vi "Line Configuration Dialog.vi"(8 "error in":errorcluster, 9 "engine configuration in":refnum<class "engine configuration.lvclass">, 10 "tag bus configurable plugin module configuration":refnum<class "PID Module 2 configuration.lvclass">, 11 "Line":T3) -> (0 "error out":errorcluster, 1 "success":bool, 2 "changed":bool, 3 "Mappings out":T2)   [LabVIEW 2015, in "PID Module 2 editor node.lvclass"]
doc: "A dialog for allowing a user to specify the values of a new line."
uses:
  PID Module 2 editor node.lvclass
  module/configuration/Line.ctl
  <vilib>/NI/Tag Bus Module Framework/channel/TBM channel.lvclass
  Mappings.ctl
  Map.ctl
  module/configuration/permissions.ctl
  <vilib>/NI/Module Execution Interface/Engine Configuration/engine configuration.lvclass
  module/configuration/PID Module 2 configuration.lvclass
  <vilib>/NI/Tag Bus/tag/tag descriptor.lvclass/tag descriptor.ctl
  <vilib>/NI/Tag Bus Module Framework/channel/TBM channel.lvclass/TBM channel.ctl
  <vilib>/NI/Configuration Framework/serializable configuration/NISE_CEF_serializable configuration.lvclass/NISE_CEF_serializable configuration.ctl
  <vilib>/NI/Tag Bus/tag/write tag name.vi
  <vilib>/NI/Tag Bus/tag/write data type.vi
  <vilib>/NI/Tag Bus Module Framework/channel/Write channel classification.vi
  <vilib>/NI/Configuration Framework/serializable configuration/Read UID.vi
  <vilib>/NI/Tag Bus/tag/read data type.vi
  <vilib>/NI/Tag Bus Module Framework/channel/Read channel classification.vi
  <vilib>/Utility/LVClass/Get LV Class Name.vi
  <vilib>/NI/Configuration Framework/error generator/NISE_error generator.vi
  <vilib>/NI/Tag Bus/tag/tag descriptor.lvclass
  <vilib>/NI/DCAF UI Toolkit/Controls/DCAF UI Elements.lvlib
panel:
  out "errors":string
  in  "Access Type":T1
  in  "Tag":i32(listbox)
  in  "Data Type":i32(listbox)
  in  "Channel Name":string
  in  "cancel":bool
  in  "ok":bool
  # "#CodeRecommended Add implementation details here. For example, a shared variable URL."
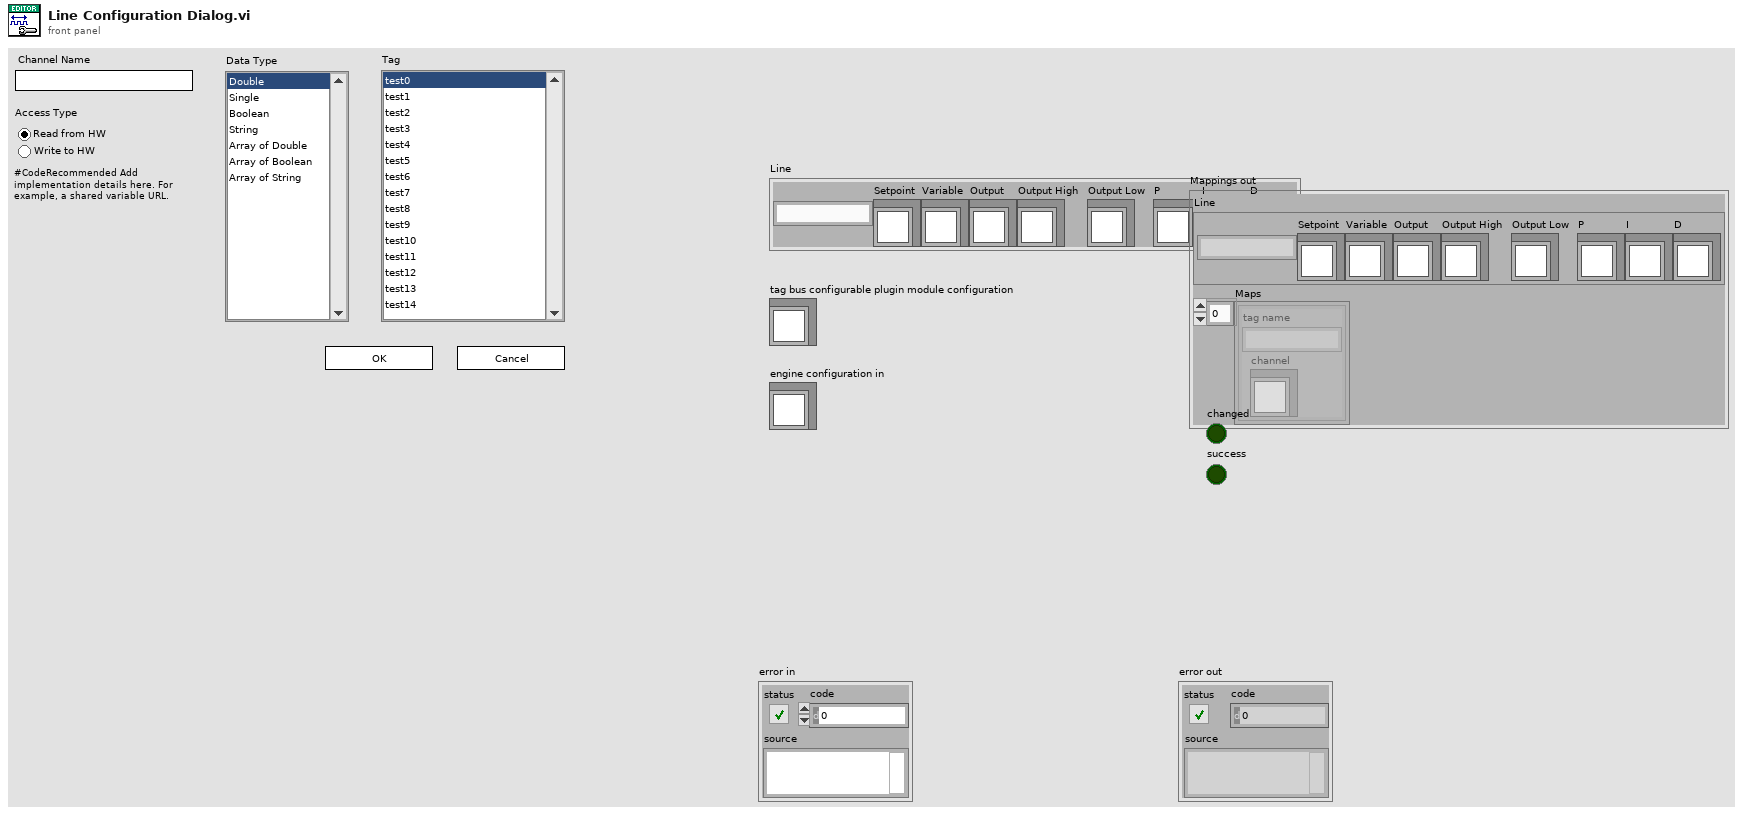
[diagram p1: front panel]
types:
  T1 = typedef "PID Module 2 configuration.lvclass/permissions.ctl" = enum32{"Read from HW", "Write to HW"}
  T2 = typedef "PID Module 2 editor node.lvclass/Mappings.ctl" = cluster{"Line":T3, "Maps":T4[]}
  T3 = typedef "PID Module 2 configuration.lvclass/Line.ctl" = cluster{"PID ID":string, "Setpoint":refnum<class "TBM channel.lvclass">, "Variable":refnum<class "TBM channel.lvclass">, "Output":refnum<class "TBM channel.lvclass">, "Output High":refnum<class "TBM channel.lvclass">, "Output Low":refnum<class "TBM channel.lvclass">, "P":refnum<class "TBM channel.lvclass">, "I":refnum<class "TBM channel.lvclass">, "D":refnum<class "TBM channel.lvclass">}
  T4 = typedef "PID Module 2 editor node.lvclass/Map.ctl" = cluster{"channel":refnum<class "TBM channel.lvclass">, "tag name":string}
  T5 = typedef "tag bus.lvlib/tag descriptor.lvclass/Data Type.ctl" = enum16{"Double", "Single", "I64", "I32", "I16", "I8", "U64", "U32", "U16", "U8", "Boolean", "String", "Array of Double", "Array of Single", "Array of I64", "Array of I32", "Array of I16", "Array of I8", "Array of U64", "Array of U32", "Array of U16", "Array of U8", "Array of Boolean", "Array of String"}
  T6 = typedef "TBM channel.lvclass/channel classification.ctl" = enum16{"input data", "output data", "processing parameter", "processing result"}
  T7 = enum8{"Enabled", "Disabled", "Disabled and Grayed Out"}
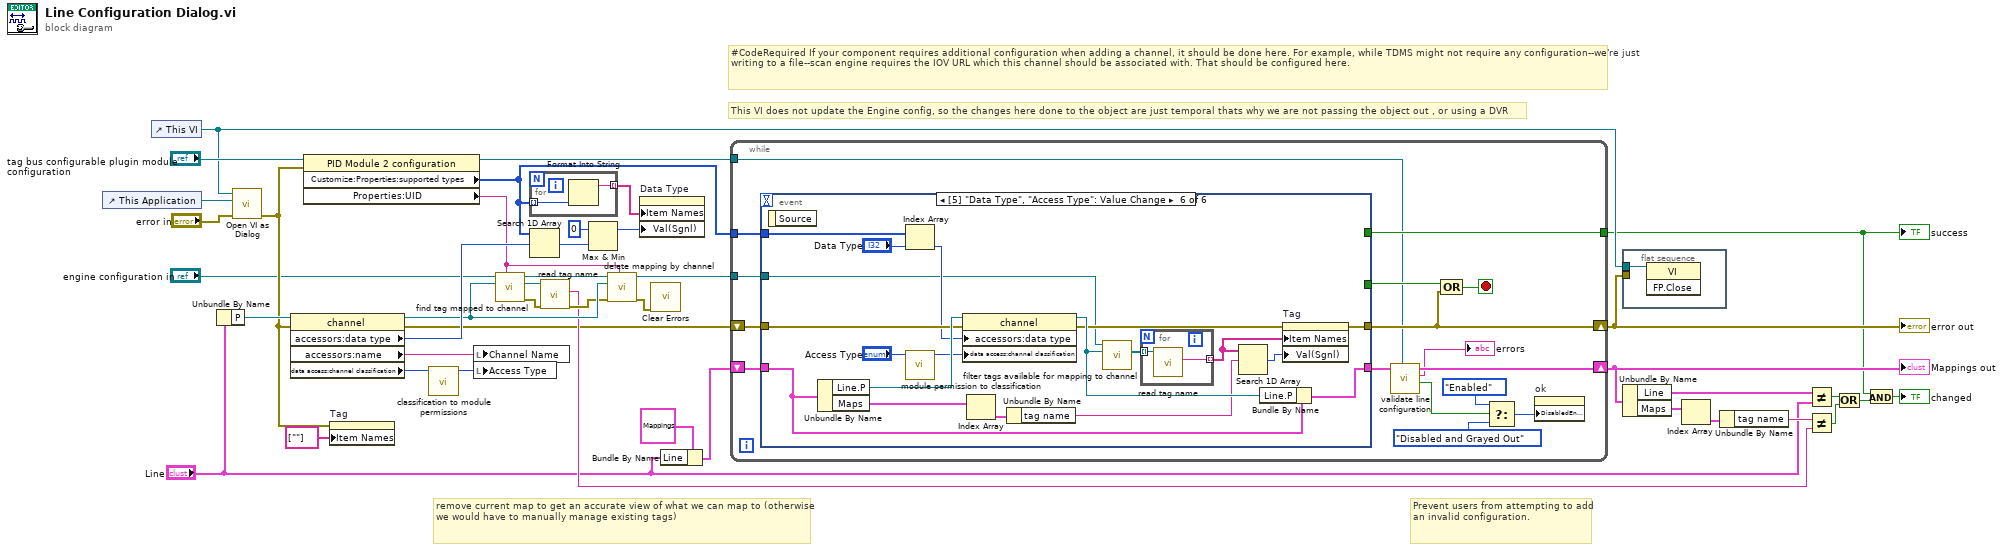
[diagram p0: block diagram]
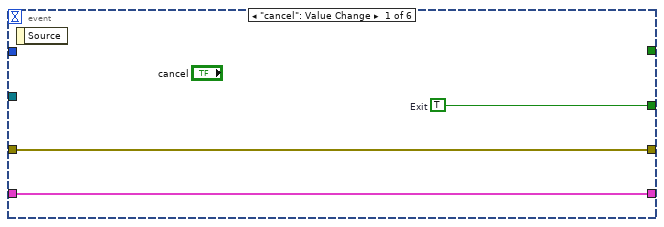
[diagram p2: hidden frame]
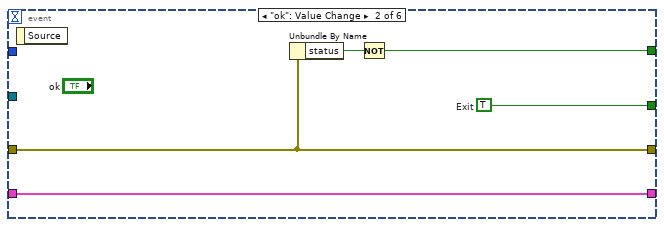
[diagram p3: hidden frame]
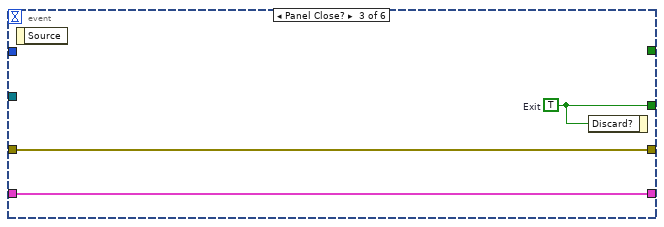
[diagram p4: hidden frame]
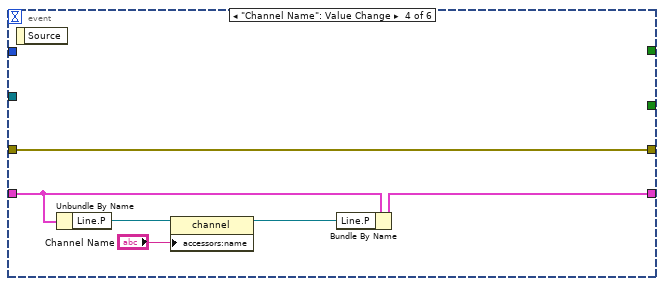
[diagram p5: hidden frame]
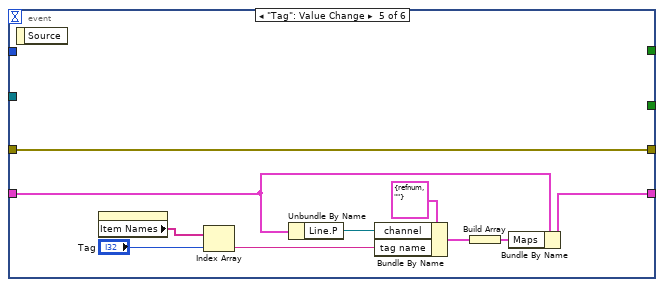
[diagram p6: hidden frame]
diagram:
  # "Prevent users from attempting to add an invalid configuration."
  # "This VI does not update the Engine config, so the changes here done to the object are just temporal thats why we are not passing the object out , or using a DVR"
  # "remove current map to get an accurate view of what we can map to (otherwise we would have to manually manage existing tags)"
  # "#CodeRequired If your component requires additional configuration when adding a channel, it should be done here. For example, while TDMS might not require any configuration--we're just writing to a file--scan engine requires the IOV URL which this channel should be associated with. That should be configured here."
  n1 = control-ref of="This Application"() -> (w31:refnum<vi>)
  n2 = control-ref of="This VI"() -> (w14:refnum<vi>)
  n3 = Unbundle By Name("Line") -> ("P"=w41:refnum<class "TBM channel.lvclass">)
  n4 = call <vilib>:"Open VI as Dialog.vi"("error in (no error)"="error in", "This Application"=w31, "VI in"=w14) -> ("error out"=w29:errorcluster)  [unwired: 8 in]
  n5 = property class="channel"(reference=w41, error in=w29) -> (reference out=w25:refnum<class "TBM channel.lvclass">, error out=w7:errorcluster, "accessors:data type"=w38:T5, "accessors:name"=w6:string, "data access:channel classification"=w8:T6)
  n6 = property class="PID Module 2 configuration"(reference="tag bus configurable plugin module configuration", error in=w29) -> (reference out=w26:refnum<class "PID Module 2 configuration.lvclass">, "Customize:Properties:supported types"=w1:T5[], "Properties:UID"=w9:string)  [unwired: 1 out]
  n7 = property on="Tag" class="LstBox (strict)"(error in=w29, "Item Names"=string[] [""]) -> ()  [unwired: 1 in, 2 out]
  n8 = call "classification to module permissions.vi"("channel classification"=w8) -> ("permissions"=w10:T1)  [unwired: 10 in]
  n9 = local write "Channel Name"(w6) -> ()
  n10 = local write "Access Type"(w10) -> ()
  n11 = call <vilib>:"find tag mapped to channel.vi"("owner"=w9, "channel"=w25, "engine configuration in"="engine configuration in") -> ("error out"=w21:errorcluster, "tag"=w22:refnum<class "tag descriptor.lvclass">, "engine configuration out"=w27:refnum<class "engine configuration.lvclass">)  [unwired: 6 in]
  n12 = for {
    tunnel: w1 -> [w44] mode=indexing
    tunnel: [w43] -> w40 mode=indexing
    n13 = Format Into String(w44) -> (resulting string=w43:string)  [unwired: 3 in, 1 out]
  }
  n14 = Search 1D Array(1D array=w1, element=w38) -> (index of element=w24:i32)  [unwired: 1 in]
  n15 = call <vilib>:"read tag name.vi"("error in"=w21, "system tag in"=w22) -> ("error out"=w20:errorcluster, "name"=w13:string)  [unwired: 7 in, 1 out]
  n16 = Max & Min(x=0 ("f"), y=w24) -> (max(x,y)=w11:i32)  [unwired: 1 out]
  n17 = call <vilib>:"delete mapping by channel.vi"("owner ID"=w9, "error in"=w20, "channel"=w25, "engine configuration in"=w27) -> ("error out"=w37:errorcluster, "engine configuration out"=w42:refnum<class "engine configuration.lvclass">)  [unwired: 6 in]
  n18 = property on="Data Type" class="LstBox (strict)"("Item Names"=w40, "Val(Sgnl)"=w11) -> ()  [unwired: 2 in, 2 out]
  n19 = call <vilib>:"Clear Errors.vi"("error in (no error)"=w37) -> ()  [unwired: 5 in, 2 out]
  n20 = Bundle By Name(cluster=T2 {"Line"={"PID ID"="", "Setpoint"=refnum, "Variable"=refnum, "Output"=refnum, "Output High"=refnum, "Output Low"=refnum, "P"=refnum, "I"=refnum, "D"=refnum}, "Maps"=[]} ("Mappings out"), "Line"="Line") -> (w34:T2)
  n21 = while {
    shift-right: [w52] -> w5
    shift-left: w7 -> [w59]
    tunnel: [w58] -> w4
    shift-right: [w53] -> w32
    shift-left: w34 -> [w55]
    tunnel: w42 -> [w60]
    tunnel: w26 -> [w47]
    tunnel: w1 -> [w46]
    stop <- w56 stop-if-true
    n22 = event shown="[5] \"Data Type\", \"Access Type\": Value Change" {
      selector: _ -> [_ _ _ _ _ _]
      dyn-events: _ -> [_ _ _ _ _ _]
      timeout: _ -> [_ _ _ _ _ _]
      tunnel: w60 -> [_ _ _ _ _ w88]
      tunnel: w59 -> [w63 w66 w71 w77 w87 w100]
      tunnel: [w63 w66 w71 w77 w87 w95] -> w52
      tunnel: [_ w64 _ _ _ _] -> w58
      tunnel: [w61 w67 w69 _ _ _] -> w57
      tunnel: w55 -> [w62 w68 w70 w75 w78 w89]
      tunnel: [w62 w68 w70 w76 w80 w103] -> w54
      tunnel: w46 -> [_ _ _ _ _ w99]
      event "cancel": Value Change {
        w61 = TRUE  # Exit
        n23 = event-data() -> ()  [unwired: 1 in, 1 out]
      }
      event "ok": Value Change {
        w67 = TRUE  # Exit
        n24 = event-data() -> ()  [unwired: 1 in, 1 out]
        n25 = Unbundle By Name(w66) -> ("status"=w65:bool)
        n26 = Not(x=w65) -> (.not. x?=w64:bool)
      }
      event Panel Close? {
        w69 = TRUE  # Exit
        n27 = event-data() -> ()  [unwired: 1 in, 1 out]
        n28 = event-data("Discard?"=w69) -> ()  [unwired: 1 in, 1 out]
      }
      event "Channel Name": Value Change {
        n29 = event-data() -> ()  [unwired: 1 in, 1 out]
        n30 = Unbundle By Name(w75) -> ("Line.P"=w74:refnum<class "TBM channel.lvclass">)
        n31 = property class="channel"(reference=w74, "accessors:name"="Channel Name") -> (reference out=w73:refnum<class "TBM channel.lvclass">)  [unwired: 1 in, 1 out]
        n32 = Bundle By Name(cluster=w75, "Line.P"=w73) -> (w76:T2)
      }
      event "Tag": Value Change {
        n33 = event-data() -> ()  [unwired: 1 in, 1 out]
        n34 = property on="Tag" class="LstBox (strict)"() -> ("Item Names"=w85:string[])  [unwired: 2 in, 2 out]
        n35 = Index Array(array=w85, index="Tag") -> (element=w79:string)
        n36 = Unbundle By Name(w78) -> ("Line.P"=w83:refnum<class "TBM channel.lvclass">)
        n37 = Bundle By Name(cluster=T4 {"channel"=refnum, "tag name"=""} ("Map"), "channel"=w83, "tag name"=w79) -> (w82:T4)
        n38 = Build Array(w82) -> (w81:T4[])
        n39 = Bundle By Name(cluster=w78, "Maps"=w81) -> (w80:T2)
      }
      event "Data Type": Value Change {
        n40 = event-data() -> ()  [unwired: 1 in, 1 out]
        n41 = Unbundle By Name(w89) -> ("Line.P"=w106:refnum<class "TBM channel.lvclass">, "Maps"=w90:T4[])
        n42 = Index Array(array=w99, index="Data Type") -> (element=w97:T5)
        n43 = call "module permission to classification.vi"("display permissions"="Access Type") -> ("channel classification"=w105:T6)  [unwired: 10 in]
        n44 = property class="channel"(reference=w106, error in=w100, "accessors:data type"=w97, "data access:channel classification"=w105) -> (reference out=w104:refnum<class "TBM channel.lvclass">, error out=w96:errorcluster)
        n45 = Index Array(array=w90) -> (element=w92:T4)  [unwired: 1 in]
        n46 = Unbundle By Name(w92) -> ("tag name"=w91:string)
        n47 = call-dynamic "filter tags available for mapping to channel.vi"("channel to map to"=w104, "engine configuration in"=w88) -> ("filtered tags"=w102:refnum<class "tag descriptor.lvclass">[])  [unwired: 8 in, 1 out]
        n48 = for {
          tunnel: w102 -> [w108] mode=indexing
          tunnel: [w107] -> w94 mode=indexing
          n49 = call <vilib>:"read tag name.vi"("system tag in"=w108) -> ("name"=w107:string)  [unwired: 8 in, 2 out]
        }
        n50 = Search 1D Array(1D array=w94, element=w91) -> (index of element=w93:i32)  [unwired: 1 in]
        n51 = Bundle By Name(cluster=w89, "Line.P"=w104) -> (w103:T2)
        n52 = property on="Tag" class="LstBox (strict)"(error in=w96, "Item Names"=w94, "Val(Sgnl)"=w93) -> (error out=w95:errorcluster)  [unwired: 1 in, 1 out]
      }
    }
    n53 = call "validate line configuration.vi"("Module Config"=w47, "Mappings in"=w54) -> ("valid?"=w51:bool, "errors"=→"errors":string, "Mappings out"=w53:T2)  [unwired: 7 in]
    n54 = Compound Arithmetic op=OR(w57, w52) -> (w56:bool)
    n55 = Select(t=T7."Enabled" ("Disabled"), s=w51, f=T7."Disabled and Grayed Out") -> (s? t:f=w48:T7)
    n56 = property on="ok" class="Bool"("DisabledEnum"=w48) -> ()  [unwired: 2 in, 2 out]
  }
  "error out" <- w5
  "success" <- w4
  "Mappings out" <- w32
  n57 = flat-sequence {
    tunnel: w5 -> [_]
    tunnel: w14 -> [w109]
    frame #0 {
      n58 = invoke class="VI" method="FP.Close"(reference=w109) -> ()  [unwired: 2 in, 3 out]
    }
  }
  n59 = Unbundle By Name(w32) -> ("Line"=w33:T3, "Maps"=w19:T4[])
  n60 = Index Array(array=w19) -> (element=w18:T4)  [unwired: 1 in]
  n61 = Unbundle By Name(w18) -> ("tag name"=w17:string)
  n62 = Not Equal?(x=w33, y="Line") -> (x != y?=w15:bool)
  n63 = Not Equal?(x=w17, y=w13) -> (x != y?=w16:bool)
  n64 = Or(x=w15, y=w16) -> (x .or. y?=w3:bool)
  n65 = And(x=w4, y=w3) -> (x .and. y?=→"changed":bool)
